vi "unload subpanel.vi"(8 "error in (no error)":errorcluster, 11 "subpanel state":T1) -> (0 "error out":errorcluster, 1 "empty?":bool, 2 "action configuration out":refnum<class "action configuration.lvclass">, 3 "subpanel state out":T1)   [LabVIEW 2014, in "Simple Sequencer TBM editor node.lvclass"]
doc: "This VI checks to see if the action VI is active. If so, it tells it to close, removes it from the subpanel, and returns its state in the configuration class."
uses:
  Simple Sequencer TBM editor node.lvclass
  subpanel state.ctl
  VI calling template typedef.ctl
  sequencer parent classes/action configuration parent/action configuration.lvclass
  user event typedef.ctl
  action config and UI pairing.ctl
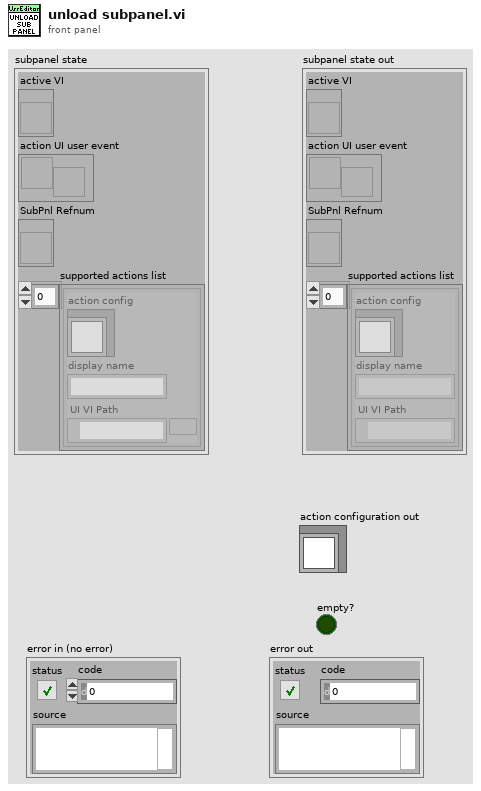
[diagram p1: front panel]
types:
  T1 = typedef "Simple Sequencer TBM editor node.lvclass/subpanel state.ctl" = cluster{"active VI":T2, "action UI user event":refnum<user-event>, "SubPnl Refnum":refnum<vi>, "supported actions list":T3[]}
  T2 = typedef "Simple Sequencer TBM editor node.lvclass/VI calling template typedef.ctl" = refnum<vi>
  T3 = typedef "Simple Sequencer TBM editor node.lvclass/action config and UI pairing.ctl" = cluster{"action config":refnum<class "action configuration.lvclass">, "display name":string, "UI VI Path":path}
  T4 = typedef "Simple Sequencer TBM editor node.lvclass/user event typedef.ctl" = cluster{"Message":string, "Data":string}
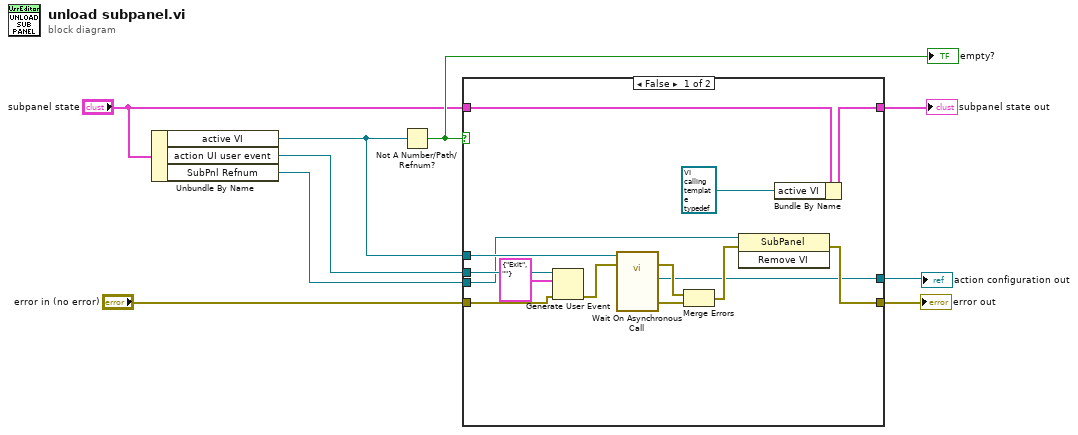
[diagram p0: block diagram]
diagram:
  n1 = Unbundle By Name("subpanel state") -> ("active VI"=w6:T2, "action UI user event"=w5:refnum<user-event>, "SubPnl Refnum"=w4:refnum<vi>)
  n2 = Not A Number/Path/Refnum?(number/path/refnum=w6) -> (NaN/Path/Refnum?=w7:bool)
  "empty?" <- w7
  n3 = case shown="False" w7 {
    tunnel: w5 -> [w23 _]
    tunnel: "error in (no error)" -> [w21 w25]
    tunnel: w6 -> [w20 _]
    tunnel: [w16 w25] -> w9
    tunnel: w4 -> [w15 _]
    tunnel: "subpanel state" -> [w13 w24]
    tunnel: [w11 w24] -> w2
    tunnel: [w10 _] -> w1
    frame False {
      n4 = Generate User Event(user event=w23, event data cluster=T4 {"Message"="Exit", "Data"=""} ("event data"), error in=w21) -> (error out=w19:errorcluster)  [unwired: 1 in, 1 out]
      n5 = call-by-ref "Wait On Asynchronous Call"(reference=w20, error in=w19) -> (error out=w18:errorcluster, 0:"error out"=w17:errorcluster, "action configuration out"=w10:refnum<class "action configuration.lvclass">)  [unwired: 10 in, 1 out]
      n6 = Merge Errors(w18, w17) -> (w14:errorcluster)
      n7 = invoke on="Invoke Node" class="SubPanel" method="Remove VI"(reference=w15, error in=w14) -> (error out=w16:errorcluster)  [unwired: 1 in, 2 out]
      n8 = Bundle By Name(cluster=w13, "active VI"=T2 refnum) -> (w11:T1)
    }
    frame True {
    }
  }
  "error out" <- w9
  "subpanel state out" <- w2
  "action configuration out" <- w1
